vi "GetFilesUSB.vi"(4 "error in (no error)":errorcluster, 6 "Test Num :":u32, 7 "Project :":string) -> (0 "error out":errorcluster, 3 "NomProjetOut":string)   [LabVIEW 2017]
uses:
  DefDeType/WhichPath.ctl
panel:
  out "Nortek File":bool
  out "Hexapod File":bool
  out "Qualisys file":bool
  out "USB file":bool
  out "Slide":u16(slide) scale=0.0..10.0
  in  "Etat":string
  # "Downloading files"
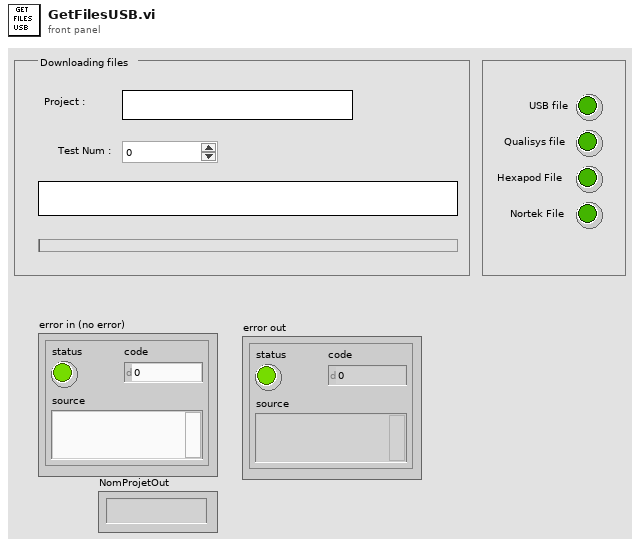
[diagram p1: front panel]
types:
  T1 = typedef "ConfigTotale.ctl" = cluster{"VoltageChannels":T2, "WheastoneBridgeChannels":T3, "Configuration":T4}
  T2 = typedef "VoltageChannels.ctl" = cluster{"ChannelNames":string[], "Sensitivity(Unit/V)":dbl[], "AutoZero":bool[], "ChannelUnits":string[], "Offsets(Units)":dbl[], "Graph Num":u8[]}
  T3 = typedef "WBridgeChannels.ctl" = cluster{"ChannelNames":string[], "Sensitivity(Unit/V)":dbl[], "AutoZero":bool[], "ChannelUnits":string[], "Offsets(Units)":dbl[], "Graph Num":u8[]}
  T4 = typedef "Configuration.ctl" = cluster{"AcqSamplingRate(Hz)":u32, "AcqTime(s)":u32, "Trigger":bool, "NbVoltageChannels":u32, "NbWBridgeChannels":u32, "Qualisys":bool, "Hexapode":bool, "FinalSamplingRate(Hz)":u32, "QualisysDataType":enum16{"6DOF", "3DTracking", "6DOF + 3D"}, "Nortek":bool, "HBM":bool}
  T5 = typedef "WhichPath.ctl" = enum16{"DossierProjet", "Config", "Meas", "MeasPCI", "MeasCRIO1", "MeasCRIO2", "MeasQualisys", "MeasHBM", "MeasTDMS", "Fig", "Res"}
  T6 = typedef "WhichPath.ctl" = enum16{"DossierProjet", "Config", "Meas", "MeasSuitCase", "MeasOnBoard", "MeasQualisys", "MeasTDMS", "MeasHexapode", "MeasNortek", "Fig", "Res", "MeasUSB"}
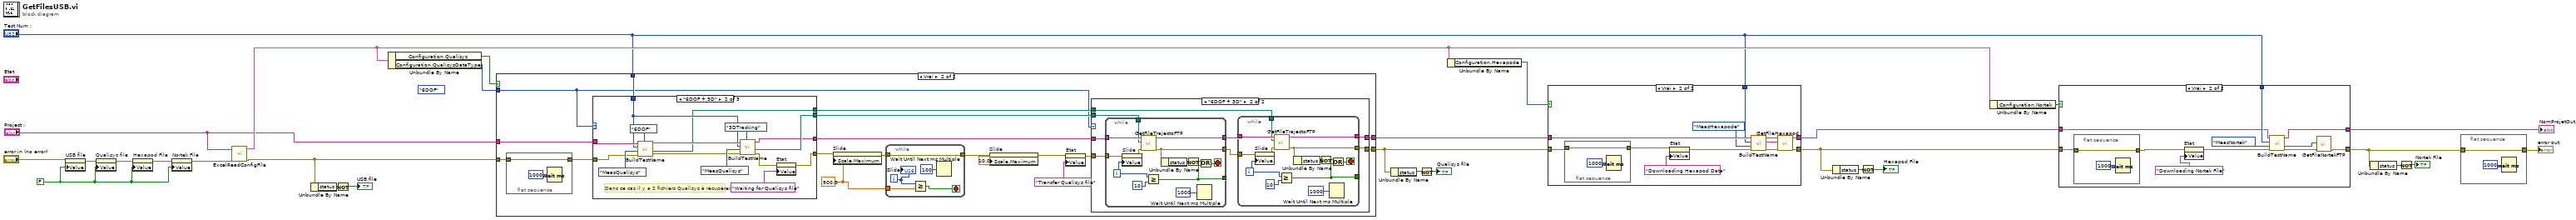
[diagram p0: block diagram]
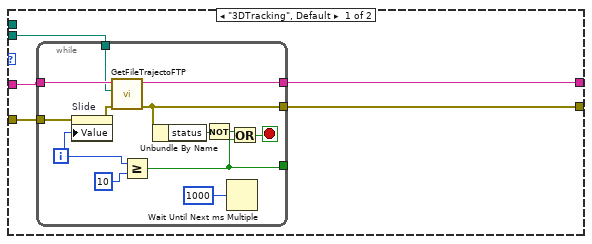
[diagram p5: hidden frame]
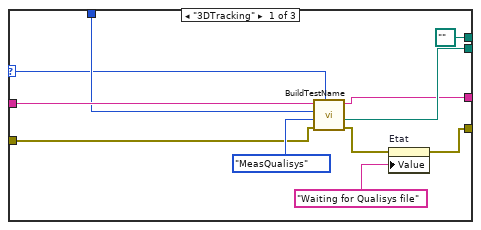
[diagram p6: hidden frame]
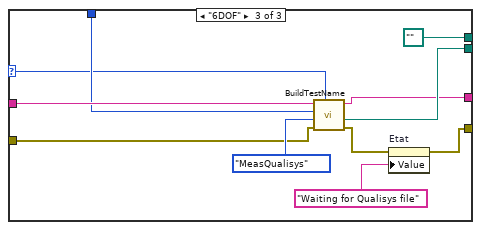
[diagram p7: hidden frame]
diagram:
  (unwired) enum16{"6DOF", "3DTracking", "6DOF + 3D"}."6DOF" ("Configuration.QualisysDataType")
  w23 = FALSE ("Valise file")
  n1 = property on="USB file" class="Bool (strict)"(error in="error in (no error)", "Value"=w23) -> (error out=w27:errorcluster)  [unwired: 1 in, 1 out]
  n2 = property on="Qualisys file" class="Bool (strict)"(error in=w27, "Value"=w23) -> (error out=w26:errorcluster)  [unwired: 1 in, 1 out]
  n3 = property on="Hexapod File" class="Bool (strict)"(error in=w26, "Value"=w23) -> (error out=w25:errorcluster)  [unwired: 1 in, 1 out]
  n4 = property on="Nortek File" class="Bool (strict)"(error in=w25, "Value"=w23) -> (error out=w24:errorcluster)  [unwired: 1 in, 1 out]
  n5 = call "ExcelReadConfigFile.vi"("NomProjet"="Project :", "error in (no error)"=w24) -> ("ConfigurationTotale"=w13:T1, "error out"=w3:errorcluster)  [unwired: 3 in]
  n6 = Unbundle By Name(w3) -> ("status"=w29:bool)
  n7 = Not(x=w29) -> (.not. x?=→"USB file":bool)
  n8 = Unbundle By Name(w13) -> ("Configuration.Qualisys"=w21:bool, "Configuration.QualisysDataType"=w1:enum16{"6DOF", "3DTracking", "6DOF + 3D"})
  n9 = case shown="Vrai" w21 {
    tunnel: w3 -> [w31 w36]
    tunnel: "Project :" -> [w30 w40]
    tunnel: w1 -> [_ w33]
    tunnel: "Test Num :" -> [_ w39]
    tunnel: [w31 w38] -> w5
    tunnel: [w30 w37] -> w18
    frame False {
    }
    frame True {
      w32 = 900.0 ("Scale.Range:Maximum")
      n10 = flat-sequence {
        tunnel: w36 -> [w140]
        tunnel: [w140] -> w35
        frame #0 {
          n11 = Wait (ms)(milliseconds to wait=u32 1000) -> ()  [unwired: 1 out]
        }
      }
      n12 = case shown="\"6DOF + 3D\"" w33 {
        selector: w33 -> [w103 _ w129]
        tunnel: [w112 w127 w138] -> w49
        tunnel: [w111 w126 w137] -> w48
        tunnel: [w110 w125 w136] -> w41
        tunnel: w40 -> [w106 w117 w132]
        tunnel: w39 -> [w105 w116 w131]
        tunnel: w35 -> [w104 w119 w130]
        tunnel: [path "" ("cheminProchainFichier") w113 path "" ("cheminProchainFichier")] -> w34
        frame "3DTracking" {
          n13 = call "BuildTestName.vi"("QualisysDataType"=w103, "entrée d'erreur"=w104, "WhichPath?"=WhichPath."MeasQualisys", "NextTestNum"=w105, "NomProjet"=w106) -> ("sortie d'erreur"=w107:errorcluster, "cheminProchainFichier"=w112:path, "NomProjetOut"=w110:string)  [unwired: 1 out]
          n14 = property on="Etat" class="Ch"(error in=w107, "Value"="Waiting for Qualisys file" ("Etat")) -> (error out=w111:errorcluster)  [unwired: 1 in, 1 out]
        }
        frame "6DOF + 3D" {
          # "Dans ce cas il y a 2 fichiers Qualisys à récupérer"
          n15 = call "BuildTestName.vi"("QualisysDataType"=enum16{"6DOF", "3DTracking"}."6DOF", "entrée d'erreur"=w119, "WhichPath?"=WhichPath."MeasQualisys", "NextTestNum"=w116, "NomProjet"=w117) -> ("sortie d'erreur"=w120:errorcluster, "cheminProchainFichier"=w113:path, "NomProjetOut"=w118:string)  [unwired: 1 out]
          n16 = call "BuildTestName.vi"("QualisysDataType"=enum16{"6DOF", "3DTracking"}."3DTracking", "entrée d'erreur"=w120, "WhichPath?"=WhichPath."MeasQualisys", "NextTestNum"=w116, "NomProjet"=w118) -> ("sortie d'erreur"=w122:errorcluster, "cheminProchainFichier"=w127:path, "NomProjetOut"=w125:string)  [unwired: 1 out]
          n17 = property on="Etat" class="Ch"(error in=w122, "Value"="Waiting for Qualisys file" ("Etat")) -> (error out=w126:errorcluster)  [unwired: 1 in, 1 out]
        }
        frame "6DOF" {
          n18 = call "BuildTestName.vi"("QualisysDataType"=w129, "entrée d'erreur"=w130, "WhichPath?"=WhichPath."MeasQualisys", "NextTestNum"=w131, "NomProjet"=w132) -> ("sortie d'erreur"=w133:errorcluster, "cheminProchainFichier"=w138:path, "NomProjetOut"=w136:string)  [unwired: 1 out]
          n19 = property on="Etat" class="Ch"(error in=w133, "Value"="Waiting for Qualisys file" ("Etat")) -> (error out=w137:errorcluster)  [unwired: 1 in, 1 out]
        }
      }
      n20 = property on="Slide" class="Gliss (strict)"(error in=w48, "Scale.Maximum"=w32) -> (error out=w47:errorcluster)  [unwired: 1 in, 1 out]
      n21 = while {
        tunnel: w47 -> [w145]
        tunnel: [w145] -> w44
        tunnel: w32 -> [w141]
        i -> [w142]
        stop <- w143 stop-if-true
        n22 = Greater Or Equal?(x=w142, y=w141) -> (x >= y?=w143:bool)
        n23 = Wait Until Next ms Multiple(millisecond multiple=u32 100) -> ()  [unwired: 1 out]
        "Slide" <- w142
      }
      n24 = property on="Slide" class="Gliss (strict)"(error in=w44, "Scale.Maximum"=10.0 ("Scale.Range:Maximum")) -> (error out=w45:errorcluster)  [unwired: 1 in, 1 out]
      n25 = property on="Etat" class="Ch"(error in=w45, "Value"="Transfer Qualisys file" ("Etat")) -> (error out=w43:errorcluster)  [unwired: 1 in, 1 out]
      n26 = case shown="\"6DOF + 3D\"" w33 {
        tunnel: w49 -> [w54 w75]
        tunnel: w43 -> [w53 w74]
        tunnel: w41 -> [w52 w73]
        tunnel: [w51 w68] -> w38
        tunnel: [w50 w72] -> w37
        tunnel: w34 -> [_ w69]
        frame "3DTracking", Default {
          n27 = while {
            tunnel: w52 -> [w62]
            tunnel: w53 -> [w59]
            tunnel: [w61] -> w50
            tunnel: [w60] -> w51
            tunnel: [w63] -> _
            tunnel: w54 -> [w55]
            i -> [w56]
            stop <- w64 stop-if-true
            n28 = property on="Slide" class="Gliss (strict)"(error in=w59, "Value"=w56) -> (error out=w58:errorcluster)  [unwired: 1 in, 1 out]
            n29 = call "GetFileTrajectoFTP.vi"("error in (no error)"=w58, "NewTrajectoFile"=w55, "NomProjet"=w62) -> ("error out"=w60:errorcluster, "NomProjetOut"=w61:string)  [unwired: 3 in]
            n30 = Greater Or Equal?(x=w56, y=10 ("x")) -> (x >= y?=w63:bool)
            n31 = Unbundle By Name(w60) -> ("status"=w66:bool)
            n32 = Not(x=w66) -> (.not. x?=w65:bool)
            n33 = Wait Until Next ms Multiple(millisecond multiple=u32 1000 ("n millisecondes")) -> ()  [unwired: 1 out]
            n34 = Or(x=w65, y=w63) -> (x .or. y?=w64:bool)
          }
        }
        frame "6DOF + 3D" {
          n35 = while {
            tunnel: w73 -> [w96]
            tunnel: w74 -> [w93]
            tunnel: [w95] -> w71
            tunnel: [w94] -> w70
            tunnel: [w97] -> _
            tunnel: w75 -> [w89]
            i -> [w90]
            stop <- w98 stop-if-true
            n36 = property on="Slide" class="Gliss (strict)"(error in=w93, "Value"=w90) -> (error out=w92:errorcluster)  [unwired: 1 in, 1 out]
            n37 = call "GetFileTrajectoFTP.vi"("error in (no error)"=w92, "NewTrajectoFile"=w89, "NomProjet"=w96) -> ("error out"=w94:errorcluster, "NomProjetOut"=w95:string)  [unwired: 3 in]
            n38 = Greater Or Equal?(x=w90, y=10 ("x")) -> (x >= y?=w97:bool)
            n39 = Unbundle By Name(w94) -> ("status"=w100:bool)
            n40 = Not(x=w100) -> (.not. x?=w99:bool)
            n41 = Wait Until Next ms Multiple(millisecond multiple=u32 1000 ("n millisecondes")) -> ()  [unwired: 1 out]
            n42 = Or(x=w99, y=w97) -> (x .or. y?=w98:bool)
          }
          n43 = while {
            tunnel: w71 -> [w83]
            tunnel: w70 -> [w80]
            tunnel: [w82] -> w72
            tunnel: [w81] -> w68
            tunnel: [w84] -> _
            tunnel: w69 -> [w76]
            i -> [w77]
            stop <- w85 stop-if-true
            n44 = property on="Slide" class="Gliss (strict)"(error in=w80, "Value"=w77) -> (error out=w79:errorcluster)  [unwired: 1 in, 1 out]
            n45 = call "GetFileTrajectoFTP.vi"("error in (no error)"=w79, "NewTrajectoFile"=w76, "NomProjet"=w83) -> ("error out"=w81:errorcluster, "NomProjetOut"=w82:string)  [unwired: 3 in]
            n46 = Greater Or Equal?(x=w77, y=10 ("x")) -> (x >= y?=w84:bool)
            n47 = Unbundle By Name(w81) -> ("status"=w87:bool)
            n48 = Not(x=w87) -> (.not. x?=w86:bool)
            n49 = Wait Until Next ms Multiple(millisecond multiple=u32 1000 ("n millisecondes")) -> ()  [unwired: 1 out]
            n50 = Or(x=w86, y=w84) -> (x .or. y?=w85:bool)
          }
        }
      }
    }
  }
  n51 = Unbundle By Name(w5) -> ("status"=w20:bool)
  n52 = Not(x=w20) -> (.not. x?=→"Qualisys file":bool)
  n53 = Unbundle By Name(w13) -> ("Configuration.Hexapode"=w17:bool)
  n54 = case shown="Vrai" w17 {
    tunnel: w5 -> [w147 w149]
    tunnel: [w147 w151] -> w4
    tunnel: [w146 w154] -> w12
    tunnel: w18 -> [w146 w158]
    tunnel: "Test Num :" -> [_ w150]
    frame False {
    }
    frame True {
      n55 = flat-sequence {
        tunnel: w149 -> [w161]
        tunnel: [w161] -> w148
        frame #0 {
          n56 = Wait (ms)(milliseconds to wait=u32 1000) -> ()  [unwired: 1 out]
        }
      }
      n57 = property on="Etat" class="Ch"(error in=w148, "Value"="Downloading Hexapod Data" ("Etat")) -> (error out=w152:errorcluster)  [unwired: 1 in, 1 out]
      n58 = call "BuildTestName.vi"("entrée d'erreur"=w152, "WhichPath?"=WhichPath."MeasHexapode", "NextTestNum"=w150, "NomProjet"=w158) -> ("sortie d'erreur"=w159:errorcluster, "NomProchainFichier"=w155:string, "NomProjetOut"=w156:string)  [unwired: 1 in, 1 out]
      n59 = call "GetFileHexapod.vi"("error in"=w159, "HexpodFileName"=w155, "Projet"=w156) -> ("error out"=w151:errorcluster, "ProjetOut"=w154:string)  [unwired: 2 in, 1 out]
    }
  }
  n60 = Unbundle By Name(w4) -> ("status"=w16:bool)
  n61 = Not(x=w16) -> (.not. x?=→"Hexapod File":bool)
  n62 = Unbundle By Name(w13) -> ("Configuration.Nortek"=w14:bool)
  n63 = case shown="Vrai" w14 {
    tunnel: w4 -> [w162 w165]
    tunnel: [w163 w167] -> w9
    tunnel: w12 -> [w163 w173]
    tunnel: "Test Num :" -> [_ w174]
    tunnel: [w162 w166] -> w7
    frame False {
    }
    frame True {
      n64 = flat-sequence {
        tunnel: w165 -> [w176]
        tunnel: [w176] -> w164
        frame #0 {
          n65 = Wait (ms)(milliseconds to wait=u32 1000) -> ()  [unwired: 1 out]
        }
      }
      n66 = property on="Etat" class="Ch"(error in=w164, "Value"="Downloading Nortek File" ("Etat")) -> (error out=w170:errorcluster)  [unwired: 1 in, 1 out]
      n67 = call "BuildTestName.vi"("entrée d'erreur"=w170, "WhichPath?"=WhichPath."MeasNortek", "NextTestNum"=w174, "NomProjet"=w173) -> ("sortie d'erreur"=w169:errorcluster, "cheminProchainFichier"=w168:path, "NomProjetOut"=w167:string)  [unwired: 1 in, 1 out]
      n68 = call "GetFileNortekFTP.vi"("error in (no error)"=w169, "NewNortekFile"=w168) -> ("error out"=w166:errorcluster)  [unwired: 4 in, 1 out]
    }
  }
  "NomProjetOut" <- w9
  n69 = Unbundle By Name(w7) -> ("status"=w10:bool)
  n70 = Not(x=w10) -> (.not. x?=→"Nortek File":bool)
  n71 = flat-sequence {
    tunnel: w7 -> [w178]
    tunnel: [w178] -> w6
    frame #0 {
      n72 = Wait (ms)(milliseconds to wait=u32 1000) -> ()  [unwired: 1 out]
    }
  }
  "error out" <- w6
